vi "411x_Volt _Chan Config Dialog.vi"(8 "error in (no error)":errorcluster, 10 "Item Ref out":T1=18446744073709551615 format="%.0x", 11 "Data Entry Limits:Maximum":dbl) -> (0 "error out":errorcluster, 1 "sense (out)":T2=1008 items=["Local"=1008, "Remote"=1009], 2 "Current Limit (out)":dbl, 3 "Initial Voltage Value (out)":dbl, 4 "Cancel (out)":bool, 5 "Number of Voltage Output Channels to Add? (out)":i16, 7 "Item Ref out":T1 format="%.0x")   [LabVIEW 2023, in "NI PXIe-411x PS Custom Device.lvlib"]
uses:
  NI PXIe-411x PS Custom Device.lvlib
  <instrlib>/niDCPower/nidcpower.llb/niDCPower Sense.ctl
  <vilib>/NI VeriStand/Custom Device API/Custom Device Item Ref.ctl
  411x_Global.vi
  <vilib>/NI VeriStand/Custom Device API/Get Item Property (Boolean).vi
  <vilib>/NI VeriStand/Custom Device API/Custom Device API.lvlib
panel:
  in  "Cancel":bool
  in  "OK Button":bool
  in  "Current Limit":dbl format="%.4f"
  in  "Initial Voltage Value":dbl
  in  "sense":T2=1008 caption="Sense" items=["Local"=1008, "Remote"=1009]
  in  "Number of Voltage Output Channels to Add?":i16=1
  # "Voltage Channels"
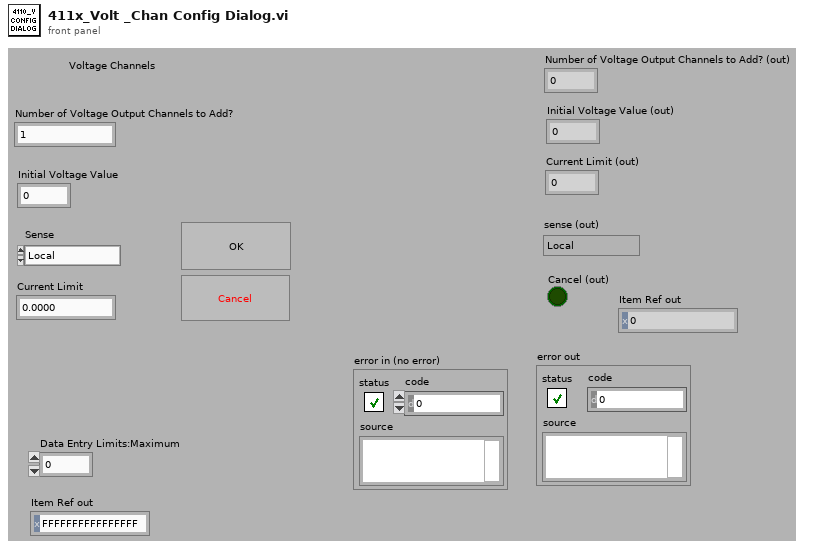
[diagram p1: front panel]
types:
  T1 = typedef "Custom Device API.lvlib/Custom Device Item Ref.ctl" = u64
  T2 = typedef "niDCPower Sense.ctl" = i32
  T3 = cluster{"V_min":dbl, "V_max":dbl, "I_min":dbl, "I_max":dbl}
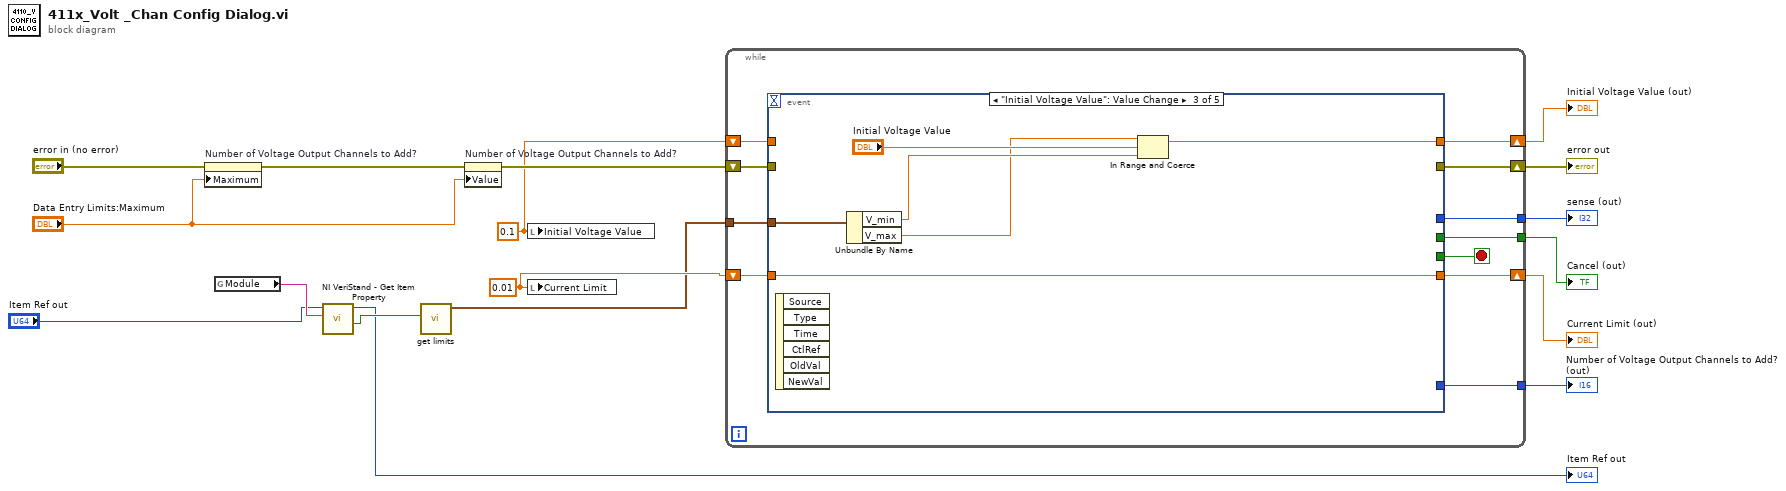
[diagram p0: block diagram]
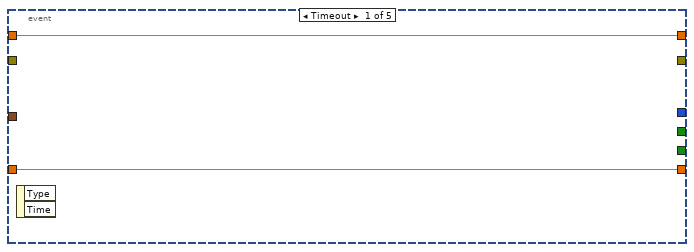
[diagram p2: hidden frame]
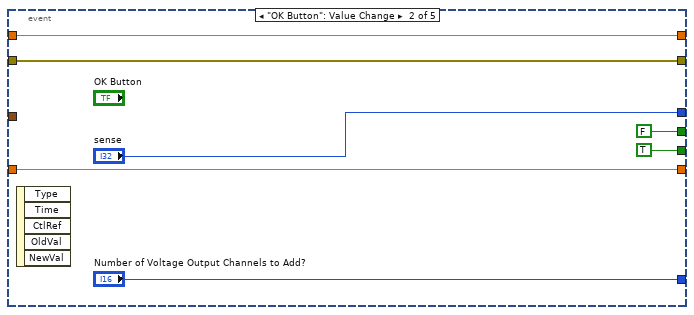
[diagram p3: hidden frame]
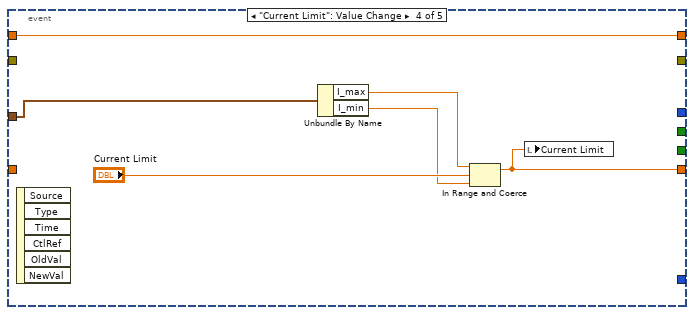
[diagram p4: hidden frame]
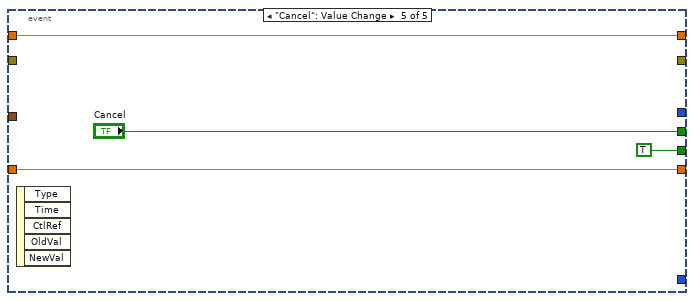
[diagram p5: hidden frame]
diagram:
  w6 = 0.1 ("Initial Voltage Value")
  w7 = 0.01 ("Current Limit")
  n1 = property on="Number of Voltage Output Channels to Add?" class="DigNum (strict)"(error in="error in (no error)", "Maximum"="Data Entry Limits:Maximum") -> (error out=w17:errorcluster)  [unwired: 1 in, 1 out]
  n2 = global read "411x_Global.vi" "Module"() -> (w4:string)
  n3 = call-poly <vilib>:"NI VeriStand - Get Item Property.vi"("Property Name"=w4, "Item Ref in"="Item Ref out") -> ("Value"=w5:bool, "Item Ref out"=→"Item Ref out":T1)  [unwired: 6 in, 2 out]
  n4 = call "get limits.vi"("4112?"=w5) -> ("output cluster"=w2:T3)  [unwired: 10 in]
  n5 = property on="Number of Voltage Output Channels to Add?" class="DigNum (strict)"(error in=w17, "Value"="Data Entry Limits:Maximum") -> (error out=w15:errorcluster)  [unwired: 1 in, 1 out]
  n6 = local write "Initial Voltage Value"(w6) -> ()
  n7 = local write "Current Limit"(w7) -> ()
  n8 = while {
    tunnel: [w25] -> w12
    tunnel: [w24] -> w10
    tunnel: [w23] -> w8
    shift-right: [w27] -> w14
    shift-left: w15 -> [w28]
    shift-right: [w26] -> w13
    shift-left: w7 -> [w21]
    shift-right: [w19] -> w11
    shift-left: w6 -> [w20]
    tunnel: w2 -> [w18]
    stop <- w22 stop-if-true
    n9 = event shown="[2] \"Initial Voltage Value\": Value Change" {
      selector: _ -> [_ _ _ _ _]
      dyn-events: _ -> [_ _ _ _ _]
      timeout: _ -> [_ _ _ _ _]
      tunnel: [w30 w32 w43 w48 w51] -> w26
      tunnel: [_ "sense" _ _ _] -> w25
      tunnel: w28 -> [_ w36 _ _ _]
      tunnel: [_ w36 _ _ _] -> w27
      tunnel: [_ FALSE ("Cancel") _ _ "Cancel"] -> w24
      tunnel: [_ "Number of Voltage Output Channels to Add?" _ _ _] -> w23
      tunnel: [_ TRUE ("Cancel") _ _ TRUE ("Cancel")] -> w22
      tunnel: w21 -> [w30 w32 w43 _ w51]
      tunnel: w20 -> [w29 w31 _ w47 w50]
      tunnel: [w29 w31 w41 w47 w50] -> w19
      tunnel: w18 -> [_ _ w40 w44 _]
      event Timeout {
        n10 = event-data() -> ()  [unwired: 1 in, 2 out]
      }
      event "OK Button": Value Change {
        n11 = event-data() -> ()  [unwired: 1 in, 5 out]
      }
      event "Initial Voltage Value": Value Change {
        n12 = event-data() -> ()  [unwired: 1 in, 6 out]
        n13 = Unbundle By Name(w40) -> ("V_min"=w39:dbl, "V_max"=w38:dbl)
        n14 = In Range and Coerce(upper limit=w38, x="Initial Voltage Value", lower limit=w39) -> (coerced(x)=w41:dbl)  [unwired: 1 out]
      }
      event "Current Limit": Value Change {
        n15 = event-data() -> ()  [unwired: 1 in, 6 out]
        n16 = Unbundle By Name(w44) -> ("I_max"=w46:dbl, "I_min"=w45:dbl)
        n17 = In Range and Coerce(upper limit=w46, x="Current Limit", lower limit=w45) -> (coerced(x)=w48:dbl)  [unwired: 1 out]
        n18 = local write "Current Limit"(w48) -> ()
      }
      event "Cancel": Value Change {
        n19 = event-data() -> ()  [unwired: 1 in, 5 out]
      }
    }
  }
  "error out" <- w14
  "Current Limit (out)" <- w13
  "sense (out)" <- w12
  "Initial Voltage Value (out)" <- w11
  "Cancel (out)" <- w10
  "Number of Voltage Output Channels to Add? (out)" <- w8
